vi "Read Result.vi"(10 "Index (0)":i32, 11 "Results in":refnum<class "Results.lvclass">) -> (2 "Result.lvclass":refnum<class "Result.lvclass">, 3 "Results out":refnum<class "Results.lvclass">)   [LabVIEW 2018, in "InfluxDB Client.lvlib" / "Results.lvclass"]
uses:
  Results.lvclass
  Result/Result.lvclass
  Results.lvclass/Results.ctl
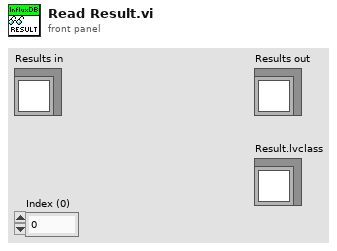
[diagram p1: front panel]
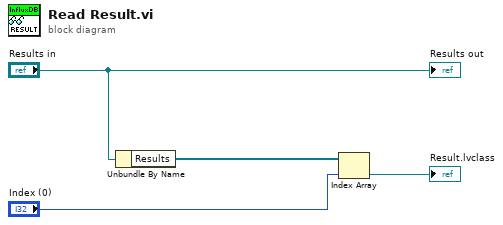
[diagram p0: block diagram]
diagram:
  n1 = Unbundle By Name("Results in") -> ("Results"=w2:refnum<class "Result.lvclass">[])
  n2 = Index Array(array=w2, index="Index (0)") -> (element=→"Result.lvclass":refnum<class "Result.lvclass">)
  "Results out" <- "Results in"
